vi "NewIndependentDigitizer.vi"() -> ()   [LabVIEW 2020]
uses:
  <vilib>/userdefined/High Color/nirio_resource_hc.ctl
  Digitizer_StatesMain.ctl
  <vilib>/Platform/TimedLoop/XDataNode/timing_clust.ctl
  <vilib>/Platform/TimedLoop/XDataNode/nitl_modes.ctl
  <vilib>/Platform/TimedLoop/XDataNode/wakeup.ctl
  <extravilib>/ChannelInstances/Stream-a[.](u16)/Read With Abort.vi
  <extravilib>/ChannelInstances/Stream-a[.](u16)/Write With Abort.vi
  <extravilib>/ChannelInstances/Stream-a[.](u16)/EndpointRead.vi
  <extravilib>/ChannelInstances/Stream-a[.](u16)/Endpoint.vi
  <extravilib>/ChannelInstances/Stream-a[.](u16)/Instantiate.vi
  <extravilib>/ChannelInstances/Stream-a[.](u16)/)Channel.vi
  <resource>/ChannelSupport/_ChannelSupport/WaitIfNeeded.vi
  <instrlib>/_niInstr/Basic Elements/v1/FPGA/Private/Count Up U32.vi
  <vilib>/FPGAPlugInAG/PXIe-7962R/niLvFpga_Open_PXIe-7962R.vi
  <vilib>/rvi/interface/common/dynamic/niFpgaDynamicAddResources.vi
  <vilib>/FPGAPlugInAG/Dynamic/niLvFpga_Close_Dynamic.vi
  <vilib>/Platform/TimedLoop/XDataNode/XDataNode.xnode
  <vilib>/rvi/interface/nirviOpenFPGA/nirviOpenFPGA.xnode
  FPGA Bitfiles/DigitizerFPGACode(Fully_Functional).lvbitx
  <vilib>/rvi/interface/nirviCloseFPGA/nirviCloseFPGA.xnode
  <instrlib>/_niInstr/Basic Elements/v1/FPGA/niInstr Basic Elements v1 FPGA.lvlib
  <vilib>/Platform/TimedLoop/XDataNode/XDNodeRunTimeDep.lvlib
  <extravilib>/ChannelInstances/Stream-a[.](u16).lvlib
  <extravilib>/ChannelInstances/Stream-a[.](i16).lvlib
panel:
  in  "reset Rx wave count":bool
  out "Waves Received":u32
  out "Digi State":T1
  in  "Stop Digi App":bool caption="Stop Digi \nApplication"
  in  "Digi Machine Mode":enum16{"Scanning Mode", "Live Mode", "Normal"}(ring)=enum."Normal"
  out "Range (Vpp)":dbl=1.3
  in  "TrigIn_Sim":bool caption="Pause"
  in  "Delay(us)":sgl min=0 step=0.1 format="%#_4g"
  in  "Record Size":u16=1024
  in  "Time Division":u8(slide)=1 max=2 step=1 scale=0.0..2.0
  in  "Amplitude \nAveraging":u16(slide)=1 caption="Amplitude Averaging" scale=0.0..7.0 scale format="%#.2g"
  out "Configured?":bool
  out "TIS Configured?":bool
  in  "Start Digi":bool
  out "Digitizer On":bool
  in  "FineDelayControl":dbl(slide)=1.0 step=0.1 scale=-2.0..2.0
  in  "Amplitude Range":cluster{"Slider 1":dbl, "Slider 1":dbl}(slide)={"Slider 1"=1.0, "Slider 1"=1.6299559471365639} scale=-2.5..2.5
  in  "Delay_Scroll_Range":dbl=2.0 caption="Range"
  out "Waveform LIVE":cluster{"Start Time":dbl, dbl, ext[]}(graph)
  in  "RIO Resource":T2="PXI1Slot2"
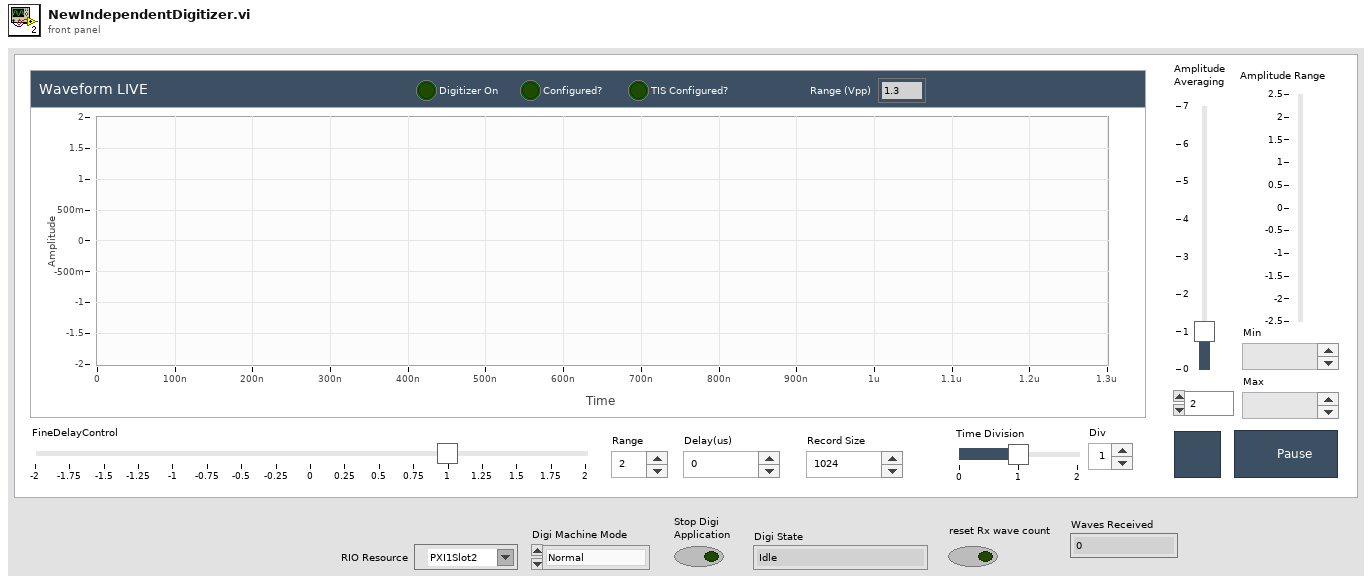
[diagram p1: front panel]
types:
  T1 = typedef "Digitizer_StatesMain.ctl" = enum16{"Idle", "Init", "SetParam", "VITrig", "Read", "CloseDigi", "CloseApp"}
  T2 = typedef "nirio_resource_hc.ctl" = tag
  T3 = typedef "XDNodeRunTimeDep.lvlib/timing_clust.ctl" = cluster{"Expected End [f-1]":u64, "Actual End [f-1]":u64, "Finished Late? [f-1]":bool, "Expected End [i-1]":u64, "Actual End [i-1]":u64, "Finished Late? [i-1]":bool, "Expected Start [i]":u64, "Actual Start [i]":u64, "Expected Start [f]":u64, "Actual Start [f]":u64, "Source Name":string, "Structure Name":string, "Period":i64, "Deadline":i64, "Offset":i64, "Start":i64, "Priority":i32, "Timeout":i32, "Mode":T4, "Wakeup Reason":T5, "Error":errorcluster, "Source Type":string, "Secondary Source Type":string, "Global End Time":u64, "Global Start Time":u64, "Frame Duration":u64, "Iteration Duration":u64, "Assigned CPU":i32, "I/O Scan Engine Mode":u32}
  T4 = typedef "XDNodeRunTimeDep.lvlib/nitl_modes.ctl" = enum32{"No Change", "Process missed periods, maintain original phase", "Discard missed periods, maintain original phase", "Process missed periods, ignore original phase", "Discard missed periods, ignore original phase"}
  T5 = typedef "XDNodeRunTimeDep.lvlib/wakeup.ctl" = enum32{"Normal", "Aborted", "Asynchronous wakeup", "Timing source error", "Timed loop error", "Timeout"}
  T6 = typedef "Stream-a[.](u16).lvlib/)Channel.ctl" = refnum<queue>
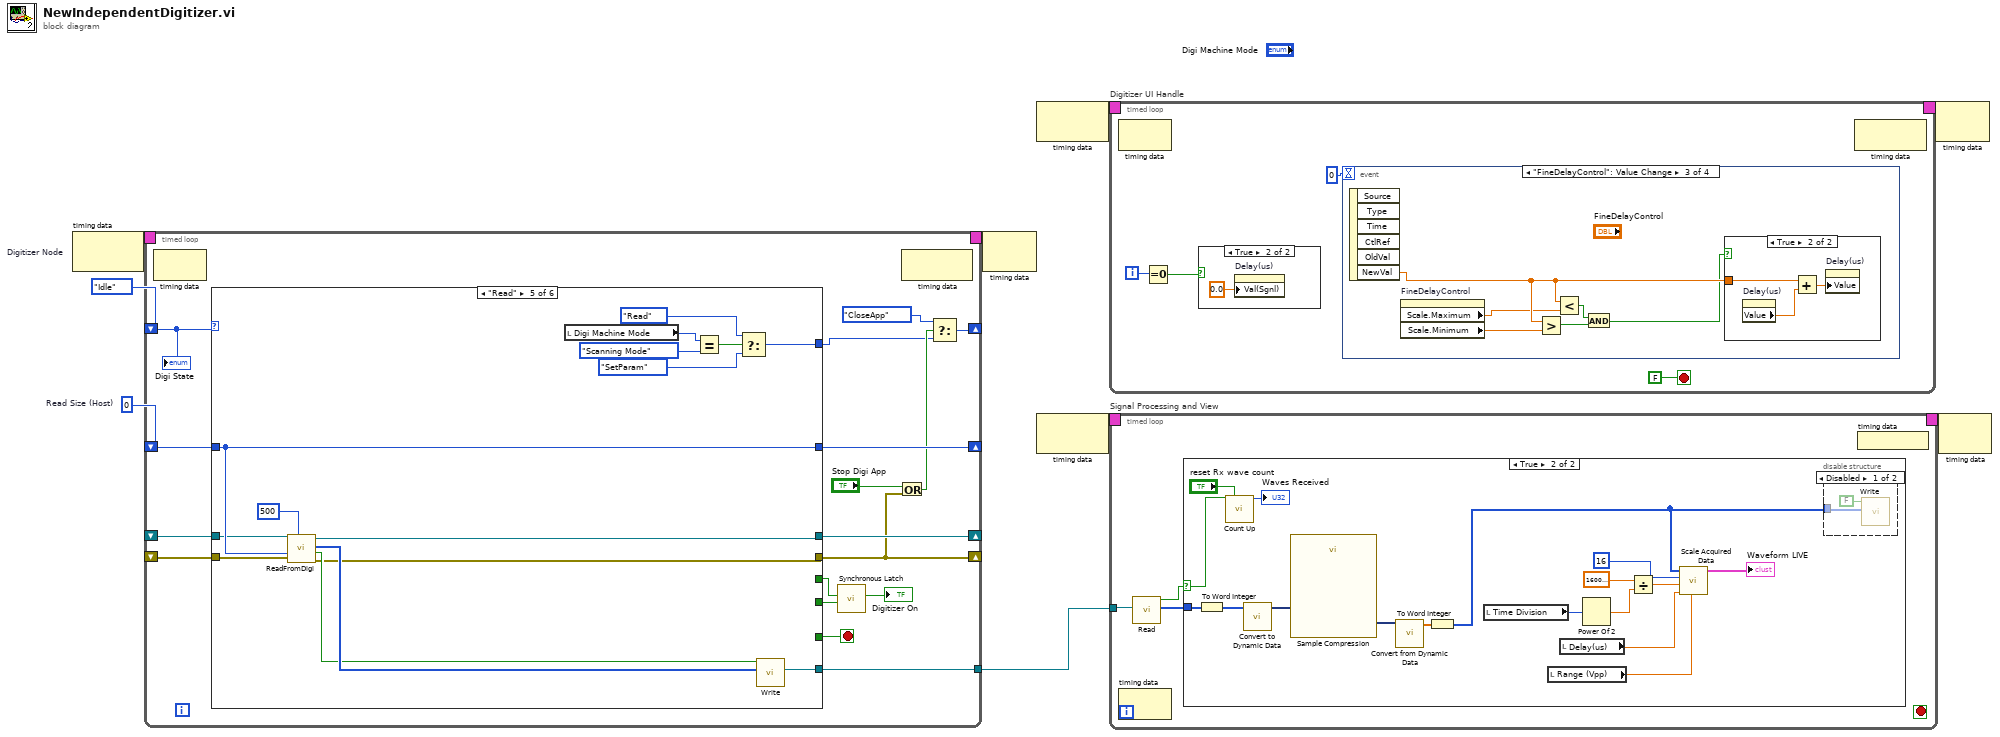
[diagram p0: block diagram]
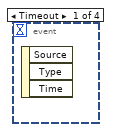
[diagram p3: hidden frame]
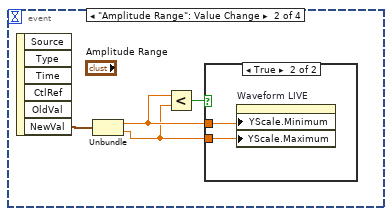
[diagram p4: hidden frame]
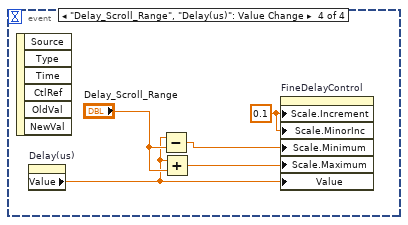
[diagram p7: hidden frame]
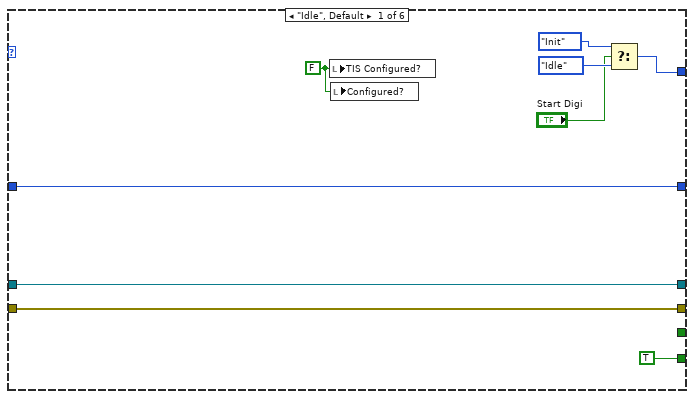
[diagram p10: hidden frame]
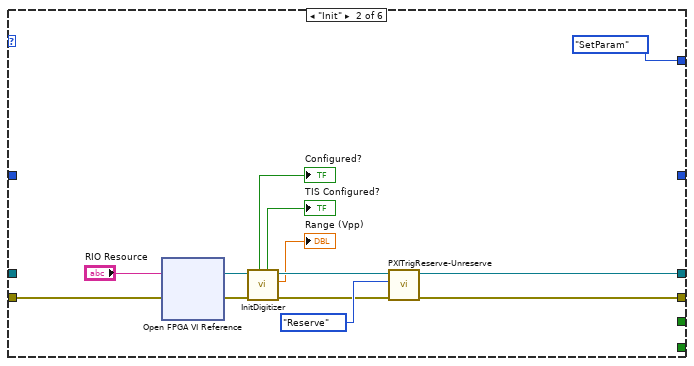
[diagram p11: hidden frame]
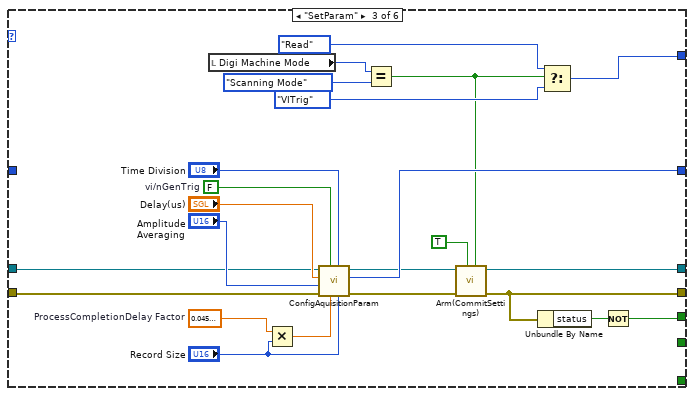
[diagram p12: hidden frame]
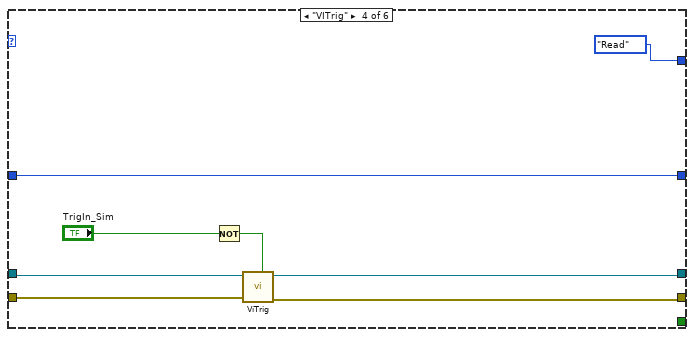
[diagram p13: hidden frame]
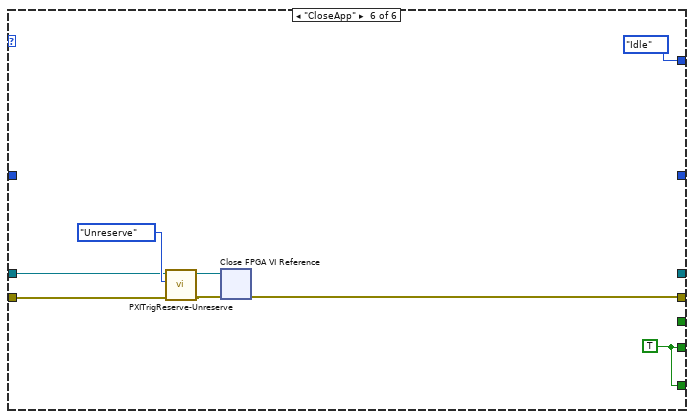
[diagram p14: hidden frame]
diagram:
  w8 = u16 0  # Read Size (Host)
  n1 = node-c288 "Digitizer Node"() -> (w7:T3)  [unwired: 1 in]
  n2 = timed-loop {
    shift-right: [w11] -> _
    shift-left: _ -> [w25]
    shift-right: [w24] -> _
    shift-left: _ -> [w23]
    shift-right: [w13] -> _
    shift-left: Digitizer_StatesMain."Idle" -> [w26]
    shift-right: [w20] -> _
    shift-left: w8 -> [w19]
    timing: w7 -> [_]
    timing-out: [_] -> w6
    tunnel: [w10] -> w3
    stop <- w17 stop-if-true
    n3 = node-c288() -> ()  [unwired: 1 in, 1 out]
    n4 = case shown="\"Read\"" w26 {
      tunnel: w25 -> [w33 w49 w73 w80 w96 w101]
      tunnel: [w33 w40 w66 w79 w82 w99] -> w11
      tunnel: [w32 w39 w56 w74 w83 _] -> w24
      tunnel: w23 -> [w32 _ w58 w75 w87 w100]
      tunnel: [w34 Digitizer_StatesMain."SetParam" ("f") w62 Digitizer_StatesMain."Read" ("f") w91 Digitizer_StatesMain."Idle" ("f")] -> w12
      tunnel: [_ _ w64 _ _ _] -> w21
      tunnel: [w31 _ w60 w76 w90 _] -> w20
      tunnel: w19 -> [w31 _ _ w76 w90 _]
      tunnel: [TRUE _ _ _ _ w98] -> w18
      tunnel: [_ _ _ _ _ w98] -> w17
      tunnel: [_ _ _ _ w88 _] -> w10
      frame "Idle", Default {
        w29 = FALSE ("TIS Configured?")
        n5 = local write "TIS Configured?"(w29) -> ()
        n6 = local write "Configured?"(w29) -> ()
        n7 = Select(t=Digitizer_StatesMain."Init", s="Start Digi", f=Digitizer_StatesMain."Idle") -> (s? t:f=w34:T1)
      }
      frame "Init" {
        n8 = xnode "Open FPGA VI Reference"("error in"=w49, "resource name"="RIO Resource") -> ("FPGA VI Reference Out"=w48:refnum<k20>, "error out"=w47:errorcluster)
        n9 = call "InitDigitizer.vi"("error in"=w47, "FPGA VI Reference In"=w48) -> ("error out"=w42:errorcluster, "range (Vpp)"=→"Range (Vpp)":dbl, "FPGA VI Reference Out"=w43:refnum<k20>, "TIS Configured?"=→"TIS Configured?":bool, "Configured?"=→"Configured?":bool)  [unwired: 5 in]
        n10 = call "PXITrigReserve-Unreserve.vi"("error in"=w42, "Mode"=enum16{"Reserve", "Unreserve"}."Reserve", "FPGA VI Reference In"=w43) -> ("error out"=w40:errorcluster, "FPGA VI Reference Out"=w39:refnum<k20>)  [unwired: 7 in]
      }
      frame "SetParam" {
        w70 = FALSE  # vi/nGenTrig
        w53 = sgl 0.045  # ProcessCompletionDelay Factor
        n11 = local read "Digi Machine Mode"() -> (w59:enum16{"Scanning Mode", "Live Mode", "Normal"})
        n12 = Multiply(x=w53, y="Record Size") -> (x*y=w52:sgl)
        n13 = call "ConfigAquisitionParam.vi"("Requested Samples Per Pixel"="Record Size", "Downsample [0,1,2]"="Time Division", "ProcessCompletionDelay (us)"=w52, "vi/nGenTrig"=w70, "error in"=w73, "AvgCount_powerOf2"="Amplitude \nAveraging", "Delay (us)"="Delay(us)", "FPGA VI Reference In"=w58) -> ("error out"=w68:errorcluster, "Read Size (Host)"=w60:u16, "FPGA VI Reference Out"=w57:refnum<k20>)  [unwired: 1 in]
        n14 = Equal?(x=w59, y=enum16{"Scanning Mode", "Live Mode", "Normal"}."Scanning Mode" ("Digi Machine Mode")) -> (x = y?=w51:bool)
        n15 = call "Arm(CommitSettings).vi"("Lvl/nPulse"=w51, "Arm?"=TRUE, "error in"=w68, "FPGA VI Reference In"=w57) -> ("error out"=w66:errorcluster, "FPGA VI Reference Out"=w56:refnum<k20>)  [unwired: 6 in]
        n16 = Unbundle By Name(w66) -> ("status"=w65:bool)
        n17 = Select(t=Digitizer_StatesMain."Read" ("f"), s=w51, f=Digitizer_StatesMain."VITrig") -> (s? t:f=w62:T1)
        n18 = Not(x=w65) -> (.not. x?=w64:bool)
      }
      frame "VITrig" {
        n19 = Not(x="TrigIn_Sim") -> (.not. x?=w81:bool)
        n20 = call "ViTrig.vi"("Vi Trigger"=w81, "error in"=w80, "FPGA VI Reference In"=w75) -> ("error out"=w79:errorcluster, "FPGA VI Reference Out"=w74:refnum<k20>)  [unwired: 7 in]
      }
      frame "Read" {
        n21 = call "ReadFromDigi.vi"("Timeout (ms)"=500, "error in"=w96, "Number of Elements"=w90, "FPGA VI Reference In"=w87) -> ("error out"=w82:errorcluster, "Data Valid?"=w86:bool, "Output Waveform"=w89:u16[], "FPGA VI Reference Out"=w83:refnum<k20>)  [unwired: 4 in]
        n22 = local read "Digi Machine Mode"() -> (w85:enum16{"Scanning Mode", "Live Mode", "Normal"})
        n23 = Equal?(x=w85, y=enum16{"Scanning Mode", "Live Mode", "Normal"}."Scanning Mode" ("Digi Machine Mode")) -> (x = y?=w94:bool)
        n24 = Select(t=Digitizer_StatesMain."Read" ("f"), s=w94, f=Digitizer_StatesMain."SetParam") -> (s? t:f=w91:T1)
        n25 = call <extravilib>:"Write.vi"("element"=w89, "element valid? (T)"=w86) -> ("channel"=w88:T6)  [unwired: 7 in, 2 out]
      }
      frame "CloseApp" {
        w98 = TRUE
        n26 = call "PXITrigReserve-Unreserve.vi"("error in"=w101, "Mode"=enum16{"Reserve", "Unreserve"}."Unreserve", "FPGA VI Reference In"=w100) -> ("error out"=w102:errorcluster, "FPGA VI Reference Out"=w103:refnum<k20>)  [unwired: 7 in]
        n27 = xnode "Close FPGA VI Reference"("FPGA VI Reference In"=w103, "error in"=w102) -> ("error out"=w99:errorcluster)
      }
    }
    n28 = call <instrlib>:"Synchronous Latch.vi"("clear"=w18, "set"=w21) -> ("out"=→"Digitizer On":bool)  [unwired: 9 in]
    n29 = Or(x="Stop Digi App", y=w11) -> (x .or. y?=w15:bool)
    n30 = node-c288() -> ()  [unwired: 1 in, 1 out]
    n31 = Select(t=Digitizer_StatesMain."CloseApp", s=w15, f=w12) -> (s? t:f=w13:T1)
    "Digi State" <- w26
  }
  n32 = node-c288(w6) -> ()  [unwired: 1 out]
  n33 = node-c288() -> (w2:T3)  [unwired: 1 in]
  n34 = node-c288() -> (w5:T3)  [unwired: 1 in]
  n35 = timed-loop "Digitizer UI Handle" {
    timing: w2 -> [_]
    timing-out: [_] -> w1
    i -> [w105]
    stop <- FALSE stop-if-true
    n36 = node-c288() -> ()  [unwired: 1 in, 1 out]
    n37 = Equal To 0?(x=w105) -> (x = 0?=w106:bool)
    n38 = case shown="True" w106 {
      frame False {
      }
      frame True {
        n39 = property on="Delay(us)" class="DigNum (strict)"("Val(Sgnl)"=sgl 0.0 ("Value (Signaling)")) -> ()  [unwired: 2 in, 2 out]
      }
    }
    n40 = event shown="[2] \"FineDelayControl\": Value Change" {
      selector: _ -> [_ _ _ _]
      dyn-events: _ -> [_ _ _ _]
      timeout: 0 -> [_ _ _ _]
      event Timeout {
        n41 = event-data() -> ()  [unwired: 1 in, 3 out]
      }
      event "Amplitude Range": Value Change {
        n42 = event-data() -> ("NewVal"=w115:cluster{"Slider 1":dbl, "Slider 1":dbl})  [unwired: 1 in, 5 out]
        n43 = Unbundle(w115) -> ("Slider 1"=w114:dbl, "Slider 1"=w113:dbl)
        n44 = Less?(x=w114, y=w113) -> (x < y?=w112:bool)
        n45 = case shown="True" w112 {
          tunnel: w114 -> [_ w117]
          tunnel: w113 -> [_ w116]
          frame False {
          }
          frame True {
            n46 = property on="Waveform LIVE" class="WFGraph (strict)"("YScale.Minimum"=w117, "YScale.Maximum"=w116) -> ()  [unwired: 2 in, 2 out]
          }
        }
      }
      event "FineDelayControl": Value Change {
        n47 = event-data() -> ("NewVal"=w122:dbl)  [unwired: 1 in, 5 out]
        n48 = property on="FineDelayControl" class="Slide (strict)"() -> ("Scale.Maximum"=w121:dbl, "Scale.Minimum"=w123:dbl)  [unwired: 2 in, 2 out]
        n49 = Greater?(x=w122, y=w123) -> (0:w119:bool)
        n50 = Less?(x=w122, y=w121) -> (x < y?=w120:bool)
        n51 = And(x=w120, y=w119) -> (x .and. y?=w118:bool)
        n52 = case shown="True" w118 {
          tunnel: w122 -> [_ w125]
          frame False {
          }
          frame True {
            n53 = property on="Delay(us)" class="DigNum (strict)"() -> ("Value"=w126:sgl)  [unwired: 2 in, 2 out]
            n54 = Add(x=w125, y=w126) -> (x+y=w124:dbl)
            n55 = property on="Delay(us)" class="DigNum (strict)"("Value"=w124) -> ()  [unwired: 2 in, 2 out]
          }
        }
      }
      event "Delay_Scroll_Range", "Delay(us)": Value Change {
        w129 = 0.1 ("Scale.Range:Increment")
        n56 = event-data() -> ()  [unwired: 1 in, 6 out]
        n57 = property on="Delay(us)" class="DigNum (strict)"() -> ("Value"=w127:sgl)  [unwired: 2 in, 2 out]
        n58 = Subtract(x=w127, y="Delay_Scroll_Range") -> (x-y=w131:dbl)
        n59 = Add(x=w127, y="Delay_Scroll_Range") -> (x+y=w130:dbl)
        n60 = property on="FineDelayControl" class="Slide (strict)"("Scale.Increment"=w129, "Scale.MinorInc"=w129, "Scale.Minimum"=w131, "Scale.Maximum"=w130, "Value"=w127) -> ()  [unwired: 2 in, 2 out]
      }
    }
    n61 = node-c288() -> ()  [unwired: 1 in, 1 out]
  }
  n62 = timed-loop "Signal Processing and View" {
    timing: w5 -> [_]
    timing-out: [_] -> w4
    tunnel: w3 -> [w134]
    stop <- _ stop-if-true
    n63 = node-c288() -> ()  [unwired: 1 in, 1 out]
    n64 = call <extravilib>:"Read.vi"("channel"=w134) -> ("element"=w133:u16[], "element valid?"=w132:bool)  [unwired: 6 in, 3 out]
    n65 = case shown="True" w132 {
      selector: w132 -> [_ w137]
      tunnel: w133 -> [_ w143]
      frame False {
      }
      frame True {
        n66 = To Word Integer(number=w143) -> (16bit integer=w142:i16[])
        n67 = call-poly <instrlib>:"Count Up.vi"("increment"=w137, "reset"="reset Rx wave count") -> ("count out"=→"Waves Received":u32)  [unwired: 13 in]
        n68 = call "Convert to Dynamic Data"("Array"=w142) -> ("Dynamic Data Type"=w141:dynamicdata)  [unwired: 3 in]
        n69 = call "Sample Compression"("Signals"=w141) -> ("Mean"=w140:dynamicdata)  [unwired: 8 in, 2 out]
        n70 = call "Convert from Dynamic Data"("Dynamic Data Type"=w140) -> ("Array"=w139:dbl[])  [unwired: 3 in]
        n71 = To Word Integer(number=w139) -> (16bit integer=w138:i16[])
        n72 = local read "Time Division"() -> (w150:u8)
        n73 = local read "Range (Vpp)"() -> (w145:dbl)
        n74 = local read "Delay(us)"() -> (w146:sgl)
        n75 = Power Of 2(x=w150) -> (2^x=w149:dbl)
        n76 = Divide(x=1600000000.0 ("Sample Rate"), y=w149) -> (x/y=w148:dbl)
        n77 = call "Scale Acquired Data.vi"("range (V)"=w145, "Start Time (us)"=w146, "Sample Rate"=w148, "Number of Bits"=i16 16, "Data In"=w138) -> ("output waveform"=→"Waveform LIVE":cluster{"Start Time":dbl, dbl, ext[]})  [unwired: 6 out]
        n78 = disable-structure shown="Disabled" {
          disable-tunnel: w138 -> [w153 _]
          frame Disabled {
            n79 = call <extravilib>:"Write.vi"("element"=w153, "element valid? (T)"=FALSE) -> ()  [unwired: 7 in, 3 out]
          }
          frame Enabled {
          }
        }
      }
    }
    n80 = node-c288() -> ()  [unwired: 1 out]
  }
  n81 = node-c288(w1) -> ()  [unwired: 1 out]
  n82 = node-c288(w4) -> ()  [unwired: 1 out]
